vi "destroyCommands.vi"(8 "error in (no error)":errorcluster, 11 "SAL_Events in":refnum<class "SAL_Events.lvclass">) -> (0 "error out":errorcluster, 3 "SAL_Events out":refnum<class "SAL_Events.lvclass">)   [LabVIEW 2016, in "SAL_Events.lvclass"]
uses:
  SAL_Events.lvclass
  SAL_Events.lvclass/SAL_Events.ctl
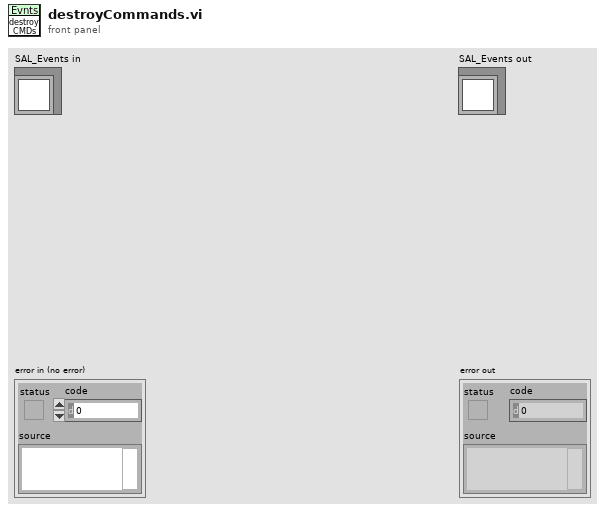
[diagram p1: front panel]
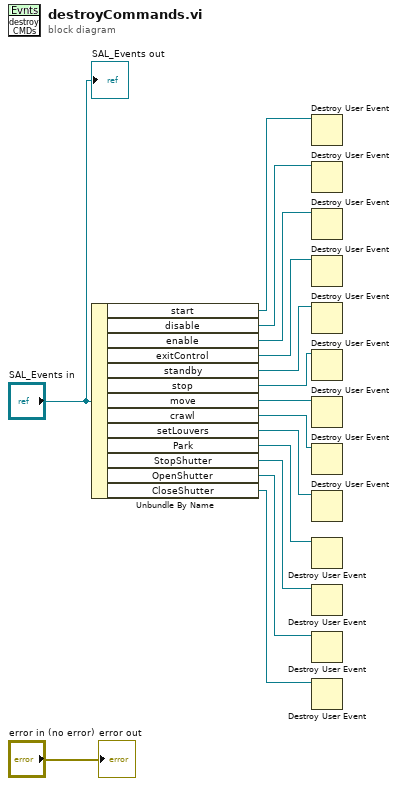
[diagram p0: block diagram]
diagram:
  n1 = Unbundle By Name("SAL_Events in") -> ("start"=w13:refnum<user-event>, "disable"=w12:refnum<user-event>, "enable"=w11:refnum<user-event>, "exitControl"=w10:refnum<user-event>, "standby"=w9:refnum<user-event>, "stop"=w8:refnum<user-event>, "move"=w7:refnum<user-event>, "crawl"=w6:refnum<user-event>, "setLouvers"=w5:refnum<user-event>, "Park"=w4:refnum<user-event>, "StopShutter"=w3:refnum<user-event>, "OpenShutter"=w2:refnum<user-event>, "CloseShutter"=w1:refnum<user-event>)
  n2 = Destroy User Event(user event=w13) -> ()  [unwired: 1 in, 1 out]
  n3 = Destroy User Event(user event=w12) -> ()  [unwired: 1 in, 1 out]
  n4 = Destroy User Event(user event=w11) -> ()  [unwired: 1 in, 1 out]
  n5 = Destroy User Event(user event=w10) -> ()  [unwired: 1 in, 1 out]
  n6 = Destroy User Event(user event=w9) -> ()  [unwired: 1 in, 1 out]
  n7 = Destroy User Event(user event=w8) -> ()  [unwired: 1 in, 1 out]
  n8 = Destroy User Event(user event=w7) -> ()  [unwired: 1 in, 1 out]
  n9 = Destroy User Event(user event=w6) -> ()  [unwired: 1 in, 1 out]
  n10 = Destroy User Event(user event=w5) -> ()  [unwired: 1 in, 1 out]
  n11 = Destroy User Event(user event=w4) -> ()  [unwired: 1 in, 1 out]
  n12 = Destroy User Event(user event=w3) -> ()  [unwired: 1 in, 1 out]
  n13 = Destroy User Event(user event=w2) -> ()  [unwired: 1 in, 1 out]
  n14 = Destroy User Event(user event=w1) -> ()  [unwired: 1 in, 1 out]
  "error out" <- "error in (no error)"
  "SAL_Events out" <- "SAL_Events in"
